vi "Status Created Events.vi"(11 "Template Queue in":refnum<class "Template Queue.lvclass">) -> (0 "Created Event Count":i32, 1 "Created Event Aliases":string[](array[string]), 2 "Created Event Exist?":bool, 3 "Template Queue out":refnum<class "Template Queue.lvclass">)   [LabVIEW 2021, in "_Template.lvlib" / "Templates.lvlib" / "Template Queue.lvlib" / "Template Queue.lvclass"]
uses:
  Template Queue.lvclass
  Template Queue.lvclass/Template Queue.ctl
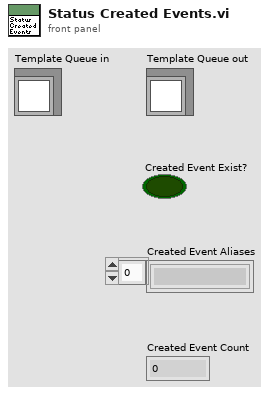
[diagram p1: front panel]
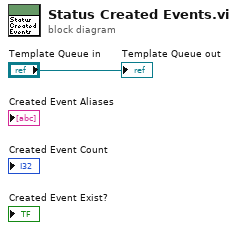
[diagram p0: block diagram]
diagram:
  "Template Queue out" <- "Template Queue in"
